vi "MGCC_MdlMgmt_main.vi"   [LabVIEW 2016]
doc: "This VI is the main VI for the model management function. The main purpose of this VI is to initize the input for the state estimation and PQ balancing. Since it will only be run one time, there is no need for the enable button."
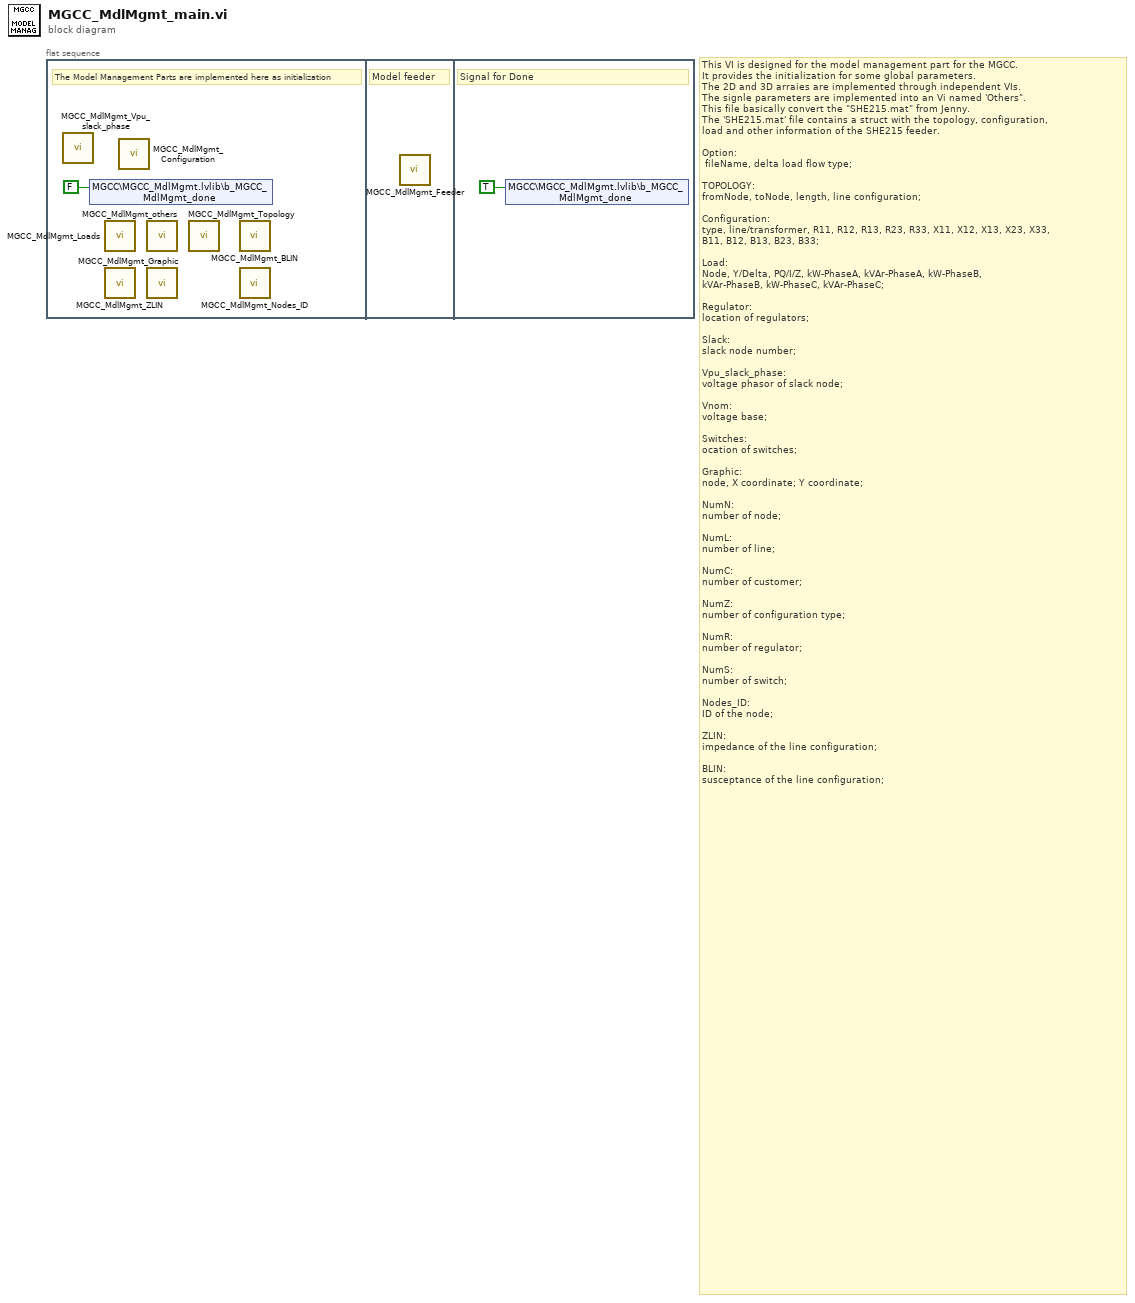
[diagram p0: block diagram]
diagram:
  # "This VI is designed for the model management part for the MGCC.\nIt provides the initialization for some global parameters.\nThe 2D and 3D arraies are implemented through independent VIs. \nThe signle parameters are implemented into an Vi named 'Others\".\nThis file basically convert the \"SHE215.mat\" from Jenny. \nThe 'SHE215.mat' file contains a struct with the topology, configuration, \nload and other information of the SHE215 feeder.\n\nOption:\n fileName, delta load flow type;\n\nTOPOLOGY:\nfromNode, toNode, length, line configuration;\n\nConfiguration: \ntype, line/transformer, R11, R12, R13, R23, R33, X11, X12, X13, X23, X33, \nB11, B12, B13, B23, B33;\n\nLoad: \nNode, Y/Delta, PQ/I/Z, kW-PhaseA, kVAr-PhaseA, kW-PhaseB, \nkVAr-PhaseB, kW-PhaseC, kVAr-PhaseC;\n\nRegulator: \nlocation of regulators;\n\nSlack: \nslack node number;\n\nVpu_slack_phase: \nvoltage phasor of slack node;\n\nVnom: \nvoltage base;\n\nSwitches: \nocation of switches;\n\nGraphic: \nnode, X coordinate; Y coordinate;\n\nNumN: \nnumber of node;\n\nNumL: \nnumber of line;\n\nNumC: \nnumber of customer;\n\nNumZ: \nnumber of configuration type;\n\nNumR: \nnumber of regulator;\n\nNumS: \nnumber of switch;\n\nNodes_ID: \nID of the node;\n\nZLIN: \nimpedance of the line configuration;\n\nBLIN: \nsusceptance of the line configuration;"
  n1 = flat-sequence {
    frame #0 {
      # "The Model Management Parts are implemented here as initialization"
      n2 = call "MGCC_MdlMgmt_Vpu_slack_phase.vi"() -> ()  [unwired: 12 in]
      n3 = shared-variable "MGCC\\MGCC_MdlMgmt.lvlib\\b_MGCC_MdlMgmt_done"(FALSE ("b_MGCC_MdlMgmt_done")) -> ()  [unwired: 1 in, 1 out]
      n4 = call "MGCC_MdlMgmt_Loads.vi"() -> ()  [unwired: 12 in]
      n5 = call "MGCC_MdlMgmt_ZLIN.vi"() -> ()  [unwired: 12 in]
      n6 = call "MGCC_MdlMgmt_Configuration.vi"() -> ()  [unwired: 12 in]
      n7 = call "MGCC_MdlMgmt_others.vi"() -> ()  [unwired: 12 in]
      n8 = call "MGCC_MdlMgmt_Graphic.vi"() -> ()  [unwired: 12 in]
      n9 = call "MGCC_MdlMgmt_Topology.vi"() -> ()  [unwired: 12 in]
      n10 = call "MGCC_MdlMgmt_BLIN.vi"() -> ()  [unwired: 12 in]
      n11 = call "MGCC_MdlMgmt_Nodes_ID.vi"() -> ()  [unwired: 12 in]
    }
    frame #1 {
      # "Model feeder"
      n12 = call "MGCC_MdlMgmt_Feeder.vi"() -> ()  [unwired: 12 in]
    }
    frame #2 {
      # "Signal for Done"
      n13 = shared-variable "MGCC\\MGCC_MdlMgmt.lvlib\\b_MGCC_MdlMgmt_done"(TRUE ("b_MGCC_MdlMgmt_done")) -> ()  [unwired: 1 in, 1 out]
    }
  }
